vi "Simulated VeriStand Engine.Allocate Channels.vi"(8 "error in (no error)":errorcluster, 11 "Simulated VeriStand Engine in":refnum<class "Simulated VeriStand Engine.lvclass">) -> (0 "error out":errorcluster, 3 "Simulated VeriStand Engine out":refnum<class "Simulated VeriStand Engine.lvclass">)   [LabVIEW 2016, in "Simulated VeriStand Engine.lvclass"]
uses:
  Simulated VeriStand Engine.lvclass
  <vilib>/NI Veristand/Custom Device API/Data Table Ref.ctl
  Simulated VeriStand Engine.lvclass/Simulated VeriStand Engine.ctl
  Simulated VeriStand Custom Device/Simulated VeriStand Custom Device.lvclass/Simulated VeriStand Custom Device.ctl
  Accessors/Read Simulated Custom Devices.vi
  Simulated VeriStand Custom Device/DSF.Simulation.Custom Device.Get Channel Count.vi
  <vilib>/NI Veristand/Custom Device API/Global Data Refs.vi
  <vilib>/NI Veristand/Custom Device API/Custom Device API.lvlib
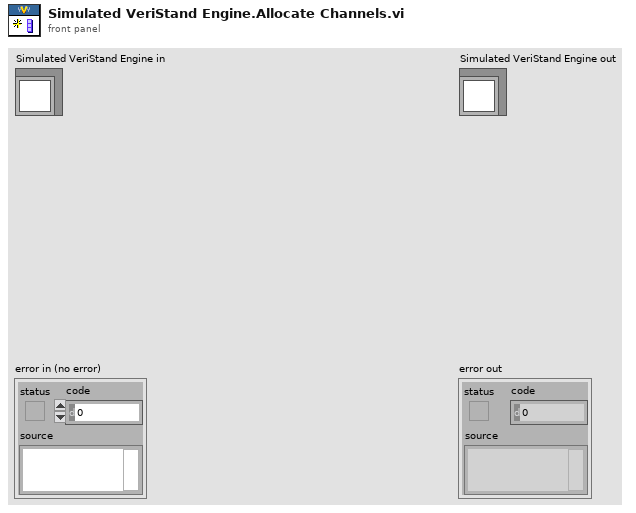
[diagram p1: front panel]
types:
  T1 = typedef "Custom Device API.lvlib/Data Table Ref.ctl" = cluster{"Ptr.Beg":u64, "Ptr.End":u64}
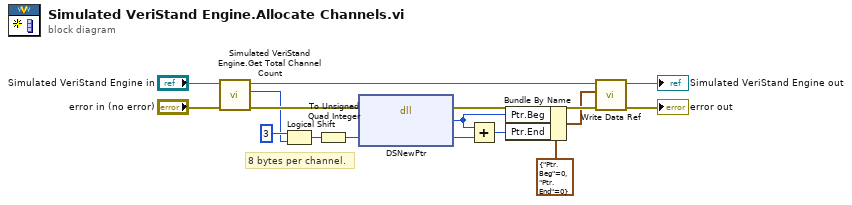
[diagram p0: block diagram]
diagram:
  # "8 bytes per channel."
  n1 = call "Simulated VeriStand Engine.Get Total Channel Count.vi"("error in (no error)"="error in (no error)", "Simulated VeriStand Engine in"="Simulated VeriStand Engine in") -> ("error out"=w5:errorcluster, "total channel count"=w2:u32, "Simulated VeriStand Engine out"=w8:refnum<class "Simulated VeriStand Engine.lvclass">)  [unwired: 7 in]
  n2 = Logical Shift(y=i16 3, x=w2) -> (x << y=w15:u32)
  n3 = To Unsigned Quad Integer(1:w15) -> (0:w10:u64)
  n4 = dll-call lib="LabVIEW" fn="DSNewPtr"(error in=w5, "size"=w10) -> (error out=w4:errorcluster, "pointer"=w11:u64, "size"=w12:u64)  [unwired: 2 in, 1 out]
  n5 = Add(x=w11, y=w12) -> (x+y=w13:u64)
  n6 = Bundle By Name(cluster=T1 {"Ptr.Beg"=0, "Ptr.End"=0} ("Data Ref"), "Ptr.Beg"=w11, "Ptr.End"=w13) -> (w1:T1)
  n7 = call "Write Data Ref.vi"("error in (no error)"=w4, "Data Table Ref"=w1, "Simulated VeriStand Engine in"=w8) -> ("error out"=→"error out":errorcluster, "Simulated VeriStand Engine out"=→"Simulated VeriStand Engine out":refnum<class "Simulated VeriStand Engine.lvclass">)  [unwired: 7 in]
